vi "Remote control temp vi.vi"() -> ()   [LabVIEW 2018]
uses:
  <vilib>/Studica/Studica Toolkit/Background/PWM Channel.ctl
panel:
  out "Position":dbl
  out "ServoGrip":bool
  out "Directions":string
  in  "stop":bool
  out "Output Distance":T1
  out "Output\nSpeed":T2
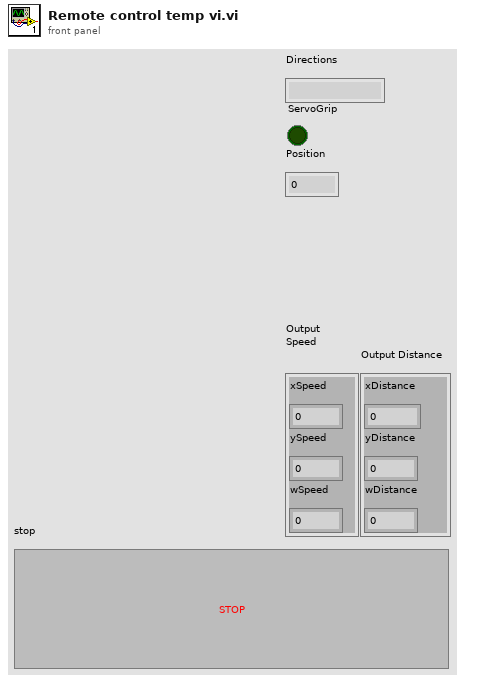
[diagram p1: front panel]
types:
  T1 = cluster{"xDistance":dbl, "yDistance":dbl, "wDistance":dbl}
  T2 = cluster{"xSpeed":dbl, "ySpeed":dbl, "wSpeed":dbl}
  T3 = typedef "PWM Channel.ctl" = enum16{"Not Connected", "A/PWM0", "A/PWM1", "A/PWM2", "A/PWM3", "A/PWM4", "B/PWM0", "B/PWM1", "B/PWM2", "B/PWM3", "B/PWM4", "C/PWM0", "C/PWM1"}
  T4 = cluster{"PWM Channel":T3, "FPGA VI Reference Out":refnum<k20>}
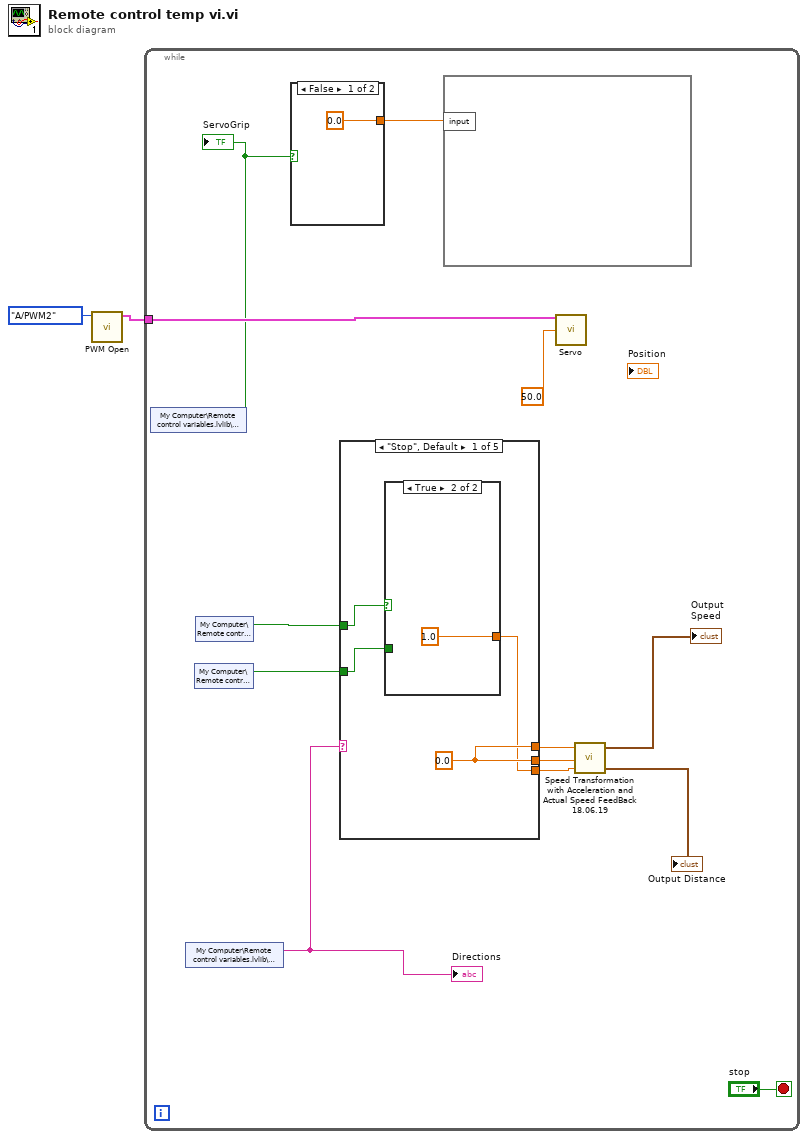
[diagram p0: block diagram]
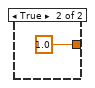
[diagram p2: hidden frame]
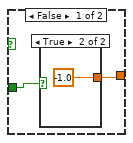
[diagram p3: hidden frame]
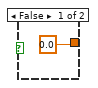
[diagram p4: hidden frame]
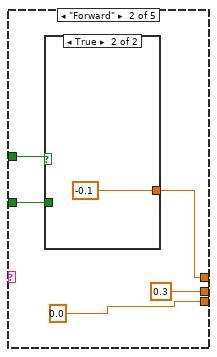
[diagram p5: hidden frame]
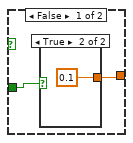
[diagram p6: hidden frame]
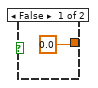
[diagram p7: hidden frame]
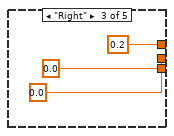
[diagram p8: hidden frame]
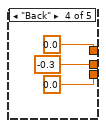
[diagram p9: hidden frame]
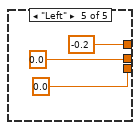
[diagram p10: hidden frame]
diagram:
  n1 = call <vilib>:"PWM Open.vi"("PWM Channel"=PWM_Channel."A/PWM2") -> ("PWM Info Out"=w1:T4)  [unwired: 9 in, 1 out]
  n2 = while {
    tunnel: w1 -> [w6]
    stop <- "stop" stop-if-true
    n3 = shared-variable "My Computer\\Remote control variables.lvlib\\ServoGrip"() -> (w4:bool)  [unwired: 1 in, 1 out]
    "ServoGrip" <- w4
    n4 = shared-variable "My Computer\\Remote control variables.lvlib\\Directions"() -> (w12:string)  [unwired: 1 in, 1 out]
    "Directions" <- w12
    n5 = shared-variable "My Computer\\Remote control variables.lvlib\\RB"() -> (w7:bool)  [unwired: 1 in, 1 out]
    n6 = shared-variable "My Computer\\Remote control variables.lvlib\\LB"() -> (w8:bool)  [unwired: 1 in, 1 out]
    n7 = case shown="False" w4 {
      tunnel: [0.0 1.0] -> w3
      frame False {
      }
      frame True {
      }
    }
    n8 = case shown="\"Stop\", Default" w12 {
      tunnel: [w19 0.3 0.0 -0.3 0.0] -> w11
      tunnel: [w19 w28 0.2 0.0 -0.2] -> w10
      tunnel: [w18 0.0 0.0 0.0 0.0] -> w9
      tunnel: w8 -> [w21 w29 _ _ _]
      tunnel: w7 -> [w20 w27 _ _ _]
      frame "Stop", Default {
        w19 = 0.0
        n9 = case shown="True" w21 {
          tunnel: [w22 1.0] -> w18
          tunnel: w20 -> [w23 _]
          frame False {
            n10 = case shown="True" w23 {
              tunnel: [0.0 -1.0] -> w22
              frame False {
              }
              frame True {
              }
            }
          }
          frame True {
          }
        }
      }
      frame "Forward" {
        n11 = case shown="True" w29 {
          tunnel: [w32 -0.1] -> w28
          tunnel: w27 -> [w33 _]
          frame False {
            n12 = case shown="True" w33 {
              tunnel: [0.0 0.1] -> w32
              frame False {
              }
              frame True {
              }
            }
          }
          frame True {
          }
        }
      }
      frame "Right" {
      }
      frame "Back" {
      }
      frame "Left" {
      }
    }
    n13 = formula code=""("input"=w3) -> ()
    n14 = call <vilib>:"Servo.vi"("PWM Info In"=w6, "Frequency [Hz]"=50.0) -> ()  [unwired: 12 in, 2 out]
    n15 = call "Speed Transformation with Acceleration and Actual Speed FeedBack 18.06.19.vi"("wTargetSpeed"=w9, "yTargetSpeed"=w11, "xTargetSpeed"=w10) -> ("Output Distance"=→"Output Distance":T1, "Output\nSpeed"=→"Output\nSpeed":T2)  [unwired: 1 in]
  }
